vi "Draw Markers.vi"(8 "error in (no error)":errorcluster, 11 "SequenceViewPanel in":refnum<class "SequenceViewPanel.lvclass">) -> (0 "error out":errorcluster, 2 "Markers":picture, 3 "SequenceViewPanel out":refnum<class "SequenceViewPanel.lvclass">)   [LabVIEW 2020, in "TSnax UI.lvlib" / "SequenceViewPanel.lvclass"]
uses:
  SequenceViewPanel.lvclass
  SequenceViewPanel.lvclass/SequenceViewPanel.ctl
  Image.ctl
  TSnax UI Manager/TSnax UI Manager.lvclass
  TSnax UI.lvlib
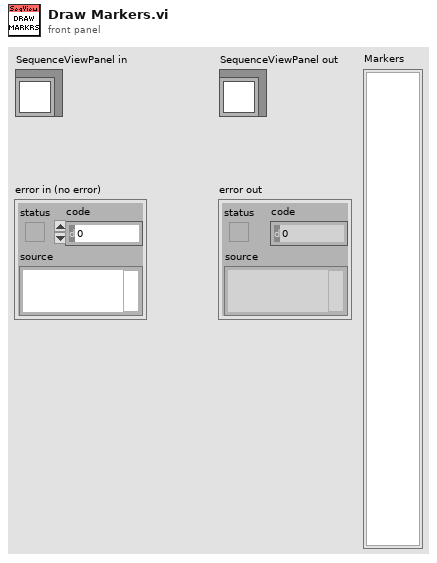
[diagram p1: front panel]
types:
  T1 = typedef "TSnax UI.lvlib/SequenceViewPanel.lvclass/Ref Data.ctl" = cluster{"Insert Index":i32, "SequenceFile":refnum<class "SequenceFile.lvclass">}
  T2 = typedef "TSnax UI.lvlib/Image.ctl" = enum16{"YellowArrow", "GreenArrow"}
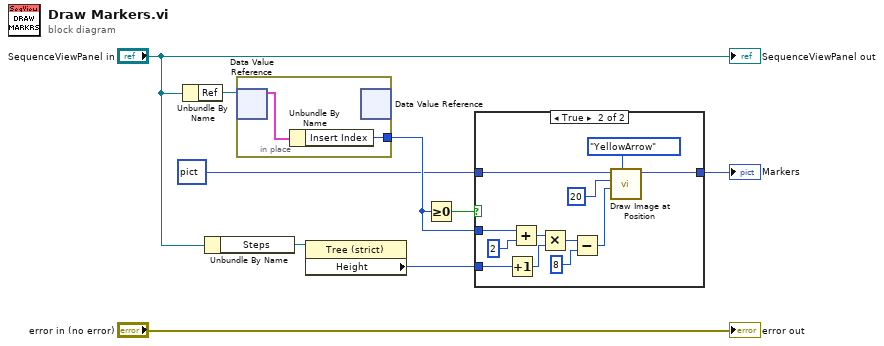
[diagram p0: block diagram]
diagram:
  n1 = Unbundle By Name("SequenceViewPanel in") -> ("Ref"=w5:refnum<data-value>)
  n2 = Unbundle By Name("SequenceViewPanel in") -> ("Steps"=w8:refnum<vi>)
  n3 = in-place {
    in-place-border: [w10] -> w3
    n4 = in-place-dvr #1(w5) -> (w11:T1)  [unwired: 1 out]
    n5 = Unbundle By Name(w11) -> ("Insert Index"=w10:i32)
    n6 = in-place-dvr #1() -> ()  [unwired: 1 in, 2 out]
  }
  n7 = property class="Tree (strict)"(reference=w8) -> ("Height"=w7:i32)  [unwired: 1 in, 2 out]
  n8 = Greater Or Equal To 0?(x=w3) -> (x >= 0?=w2:bool)
  n9 = case shown="True" w2 {
    tunnel: w7 -> [_ w17]
    tunnel: [w12 w16] -> w6
    tunnel: w3 -> [_ w15]
    tunnel: picture data[5B] ("Picture") -> [w12 w14]
    frame False {
    }
    frame True {
      n10 = Increment(x=w17) -> (x+1=w13:i32)
      n11 = Add(x=w15, y=2) -> (x+y=w22:i32)
      n12 = Multiply(x=w22, y=w13) -> (x*y=w20:i32)
      n13 = Subtract(x=w20, y=8) -> (x-y=w18:i32)
      n14 = call "Draw Image at Position.vi"("Image"=Image."YellowArrow", "Top"=w18, "Left"=i16 20, "Picture In"=w14) -> ("Picture"=w16:picture)  [unwired: 7 in]
    }
  }
  "Markers" <- w6
  "error out" <- "error in (no error)"
  "SequenceViewPanel out" <- "SequenceViewPanel in"
